vi "Stop Thread.vi"(8 "error in (no error)":errorcluster, 11 "Thread in":refnum<class "Thread.lvclass">) -> (0 "error out":errorcluster, 3 "Thread out":refnum<class "Thread.lvclass">)   [LabVIEW 2017, in "DSF Core.lvlib" / "Thread.lvclass"]
uses:
  Thread.lvclass
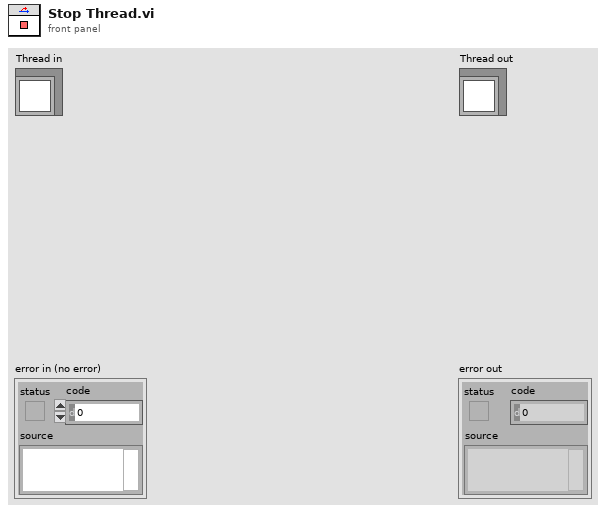
[diagram p1: front panel]
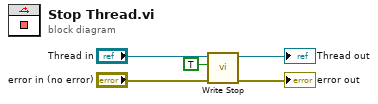
[diagram p0: block diagram]
diagram:
  n1 = call "Write Stop.vi"("error in (no error)"="error in (no error)", "stop"=TRUE, "Thread in"="Thread in") -> ("error out"=→"error out":errorcluster, "Thread out"=→"Thread out":refnum<class "Thread.lvclass">)  [unwired: 7 in]
